vi "Close_all_notifiers.vi"(10 "Process Queue Refnum array":refnum<queue>[](array[refnum]), 11 "Process Notifier Refnum array":refnum<notifier>[](array[refnum])) -> ()   [LabVIEW 2017, in "labview-standard-library.lvlib" / "automode-scripting.lvlib"]
uses:
  automode-scripting.lvlib
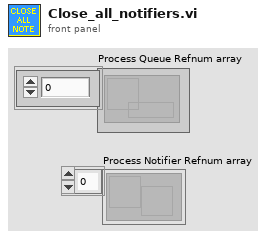
[diagram p1: front panel]
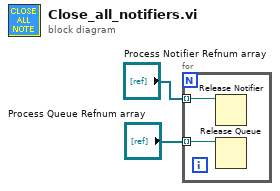
[diagram p0: block diagram]
diagram:
  n1 = for {
    tunnel: "Process Notifier Refnum array" -> [w4] mode=indexing
    tunnel: "Process Queue Refnum array" -> [w3] mode=indexing
    n2 = Release Notifier(notifier=w4) -> ()  [unwired: 2 in, 3 out]
    n3 = Release Queue(queue=w3) -> ()  [unwired: 2 in, 3 out]
  }
